vi "Save Data.vi"(8 "error in (no error)":errorcluster, 9 "Dimming Options":T1, 10 "Array of Measurements":string[][][](array[string]), 11 "Excel Saver in":refnum<class "Excel Saver.lvclass">) -> (0 "error out":errorcluster, 3 "Excel Saver out":refnum<class "Excel Saver.lvclass">)   [LabVIEW 2016, in "Data Saving.lvlib" / "Excel Saver.lvclass"]
uses:
  Excel Saver.lvclass
  Focal Point End Of Line Tester/Controls/Dimming Options.ctl
  <vilib>/Utility/NIReport.llb/NI_report.lvclass
  <vilib>/Utility/NIReport.llb/Excel/NI_Excel.lvclass
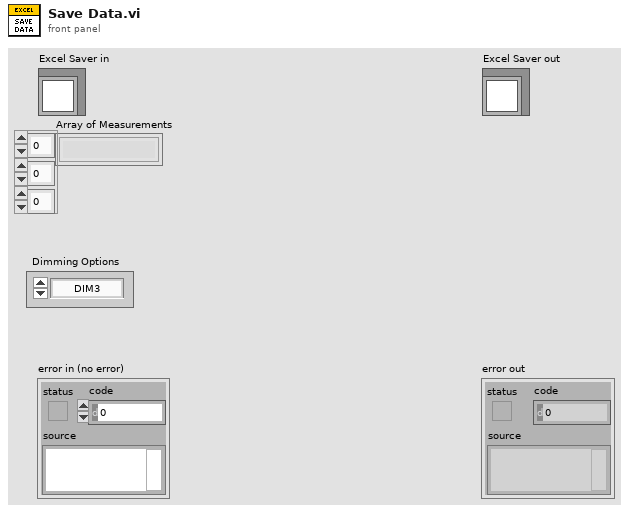
[diagram p1: front panel]
types:
  T1 = typedef "Dimming Options.ctl" = enum16{"DIM3", "DIM2", "DIM1", "NONE"}
  T2 = enum16{"Standard Report", "HTML", "Word", "Excel"}
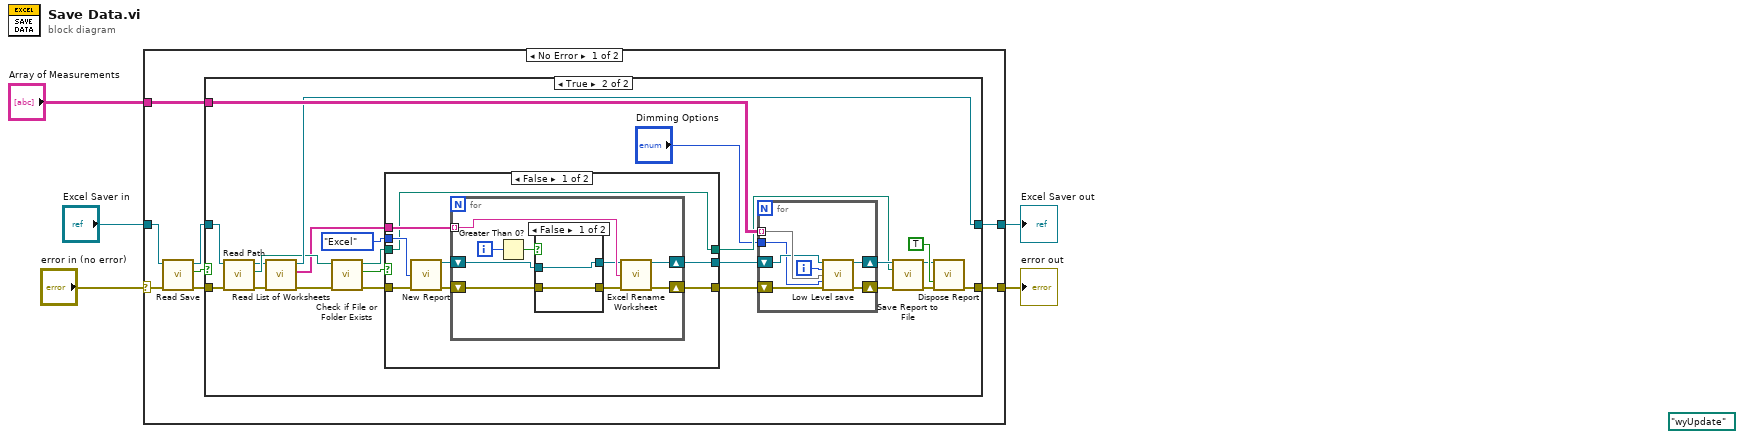
[diagram p0: block diagram]
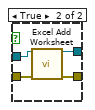
[diagram p3: hidden frame]
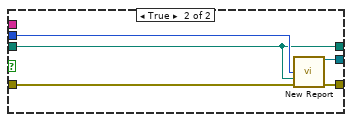
[diagram p4: hidden frame]
diagram:
  (unwired) path "wyUpdate" ("Path")
  n1 = case shown="No Error" "error in (no error)" {
    selector: "error in (no error)" -> [w9 w75]
    tunnel: [w12 w75] -> w4
    tunnel: [w11 w74] -> w2
    tunnel: "Excel Saver in" -> [w10 w74]
    tunnel: "Array of Measurements" -> [w13 _]
    frame No Error {
      n2 = call-dynamic "Read Save.vi"("error in (no error)"=w9, "Excel Saver in"=w10) -> ("error out"=w8:errorcluster, "Save"=w6:bool, "Excel Saver out"=w7:refnum<class "Excel Saver.lvclass">)  [unwired: 7 in]
      n3 = case shown="True" w6 {
        tunnel: w13 -> [_ w38]
        tunnel: [w14 w37] -> w12
        tunnel: [w15 w36] -> w11
        tunnel: w8 -> [w14 w17]
        tunnel: w7 -> [w15 w16]
        frame False {
        }
        frame True {
          n4 = call-dynamic "Read Path.vi"("error in (no error)"=w17, "Abstract Saver in"=w16) -> ("error out"=w31:errorcluster, "Path"=w35:path, "Abstract Saver out"=w32:refnum<class "Excel Saver.lvclass">)  [unwired: 7 in]
          n5 = call-dynamic "Read List of Worksheets.vi"("error in (no error)"=w31, "Excel Saver in"=w32) -> ("error out"=w30:errorcluster, "List of Worksheets"=w29:string[], "Excel Saver out"=w36:refnum<class "Excel Saver.lvclass">)  [unwired: 7 in]
          n6 = call <vilib>:"Check if File or Folder Exists.vi"("error in (no error)"=w30, "path"=w35) -> ("error out"=w33:errorcluster, "file or folder exists?"=w19:bool, "dup path"=w28:path)  [unwired: 7 in]
          n7 = case shown="False" w19 {
            tunnel: [w48 w70] -> w27
            tunnel: w33 -> [w53 w72]
            tunnel: [w47 w71] -> w26
            tunnel: T2."Excel" ("report type") -> [w52 w73]
            tunnel: w29 -> [w51 _]
            tunnel: w28 -> [w46 w69]
            tunnel: [w46 w69] -> w21
            frame False {
              n8 = call <vilib>:"New Report.vi"("report type"=w52, "error in (no error)"=w53) -> ("report out"=w50:refnum<class "NI_report.lvclass">, "error out"=w49:errorcluster)  [unwired: 12 in]
              n9 = for {
                tunnel: w51 -> [w62] mode=indexing
                shift-right: [w54] -> w48
                shift-left: w50 -> [w59]
                shift-right: [w55] -> w47
                shift-left: w49 -> [w57]
                i -> [w61]
                n10 = Greater Than 0?(x=w61) -> (x > 0?=w60:bool)
                n11 = case shown="False" w60 {
                  tunnel: w59 -> [w64 w68]
                  tunnel: [w64 w67] -> w58
                  tunnel: w57 -> [w63 w66]
                  tunnel: [w63 w65] -> w56
                  frame False {
                  }
                  frame True {
                    n12 = call <vilib>:"Excel Add Worksheet.vi"("report in"=w68, "error in (no error)"=w66) -> ("report out"=w67:refnum<class "NI_report.lvclass">, "error out"=w65:errorcluster)  [unwired: 12 in]
                  }
                }
                n13 = call <vilib>:"Excel Rename Worksheet.vi"("report in"=w58, "worksheet name (\"\")"=w62, "error in (no error)"=w56) -> ("report out"=w54:refnum<class "NI_report.lvclass">, "error out"=w55:errorcluster)  [unwired: 11 in]
              }
            }
            frame True {
              n14 = call <vilib>:"New Report.vi"("report type"=w73, "template (empty)"=w69, "error in (no error)"=w72) -> ("report out"=w70:refnum<class "NI_report.lvclass">, "error out"=w71:errorcluster)  [unwired: 11 in]
            }
          }
          n15 = for {
            tunnel: w38 -> [w45] mode=indexing
            shift-right: [w41] -> w22
            shift-left: w27 -> [w43]
            shift-right: [w40] -> w20
            shift-left: w26 -> [w42]
            tunnel: "Dimming Options" -> [w39]
            i -> [w44]
            n16 = call "Low Level save.vi"("NI_report in"=w43, "worksheet index (0)"=w44, "Array"=w45, "Dimming Options"=w39, "error in (no error)"=w42) -> ("NI_report out"=w41:refnum<class "NI_report.lvclass">, "error out"=w40:errorcluster)  [unwired: 6 in, 3 out]
          }
          n17 = call-dynamic "Save Report to File.vi"("report in"=w22, "report file path"=w21, "error in (no error)"=w20) -> ("report out"=w23:refnum<class "NI_report.lvclass">, "error out"=w25:errorcluster)  [unwired: 2 in, 9 out]
          n18 = call-dynamic "Dispose Report.vi"("report in"=w23, "save changes? (F)"=TRUE, "error in (no error)"=w25) -> ("error out"=w37:errorcluster)  [unwired: 2 in, 10 out]
        }
      }
    }
    frame Error {
    }
  }
  "error out" <- w4
  "Excel Saver out" <- w2
